vi "BioDaq_labview.vi"() -> ()   [LabVIEW 2013]
doc: "This example performs writes and reads on a serial port, as directed by the user. You can press the Write and Read buttons, and change the Read Count, while the example is running.\n\nThe parameters set for the serial port must match the parameters of the connected instrument or device. In this example, the Read Count parameter specifies the number of bytes that the serial port reads. If there were more bytes at the port than the specified number, those bytes would not be read. If there were less bytes at the port than the specified number, you would receive a timeout error.\n\nThis example expands upon the flow control options for XON and XOFF, allowing the user to choose those control characters. Also, the user can enable or disable a termination character. Some devices require a termination character in order to identify the end of command strings. Some devices send a termination character to signify the end of data to be read. This example shows how you can end the Read operation once a termination character is detected in the buffer and/or append a termination character at the end of the Write data."
uses:
  Program Files/National Instruments/LabVIEW 2013/examples/Instrument IO/Serial/support/Serial - Settings.ctl
  <vilib>/Instr/_visa.llb/VISA Configure Serial Port (Instr).vi
panel:
  in  "Write 8":bool
  in  "Write 7":bool
  in  "Write 6":bool
  in  "Write 5":bool
  out "device 4":bool
  out "device 3":bool
  out "Waveform Chart 9":T1(graph)
  out "Waveform Chart 8":T1(graph)
  out "Waveform Chart 7":T1(graph)
  out "unit type 3":dbl
  out "time3":dbl
  in  "Write 4":bool
  in  "Write 3":bool
  out "goniometer":u8(knob) scale=0.0..255.0
  out "unit type":dbl
  out "Waveform Chart 6":T1(graph)
  out "Waveform Chart 5":T1(graph)
  out "Waveform Chart 4":T1(graph)
  out "unit type 2":dbl
  out "time 2":dbl
  out "device 2":bool
  out "device 1":bool
  out "time":dbl
  in  "Write 2":bool
  out "Waveform Chart 3":T1(graph)
  out "Waveform Chart 2":T1(graph)
  out "Waveform Chart":T1(graph)
  in  "Stop":bool
  in  "Command":string="*IDN?"
  in  "Write":bool
  in  "Serial Settings":T2={"baud rate"=115200, "data bits"=8, "parity"=enum."None", "stop bits"=10, "flow control"=0} {"flow control" items=["None"=0, "XON/XOFF"=1, "RTS/CTS"=2, "DTR/DSR"=4]; "stop bits" items=["1.0"=10, "1.5"=15, "2.0"=20]; "data bits" min=5 max=8 step=1; "baud rate" items=["75"=75, "110"=110, "134"=134, "150"=150, "300"=300, "600"=600, "1200"=1200, "1800"=1800, "2400"=2400, "4800"=4800, "7200"=7200, "9600"=9600, "14400"=14400, "19200"=19200, "28800"=28800, "38400"=38400, "56000"=56000, "57600"=57600, "115200"=115200, "128000"=128000, "230400"=230400]}
  in  "VISA resource name":refnum<visa-resource-name>="COM4"
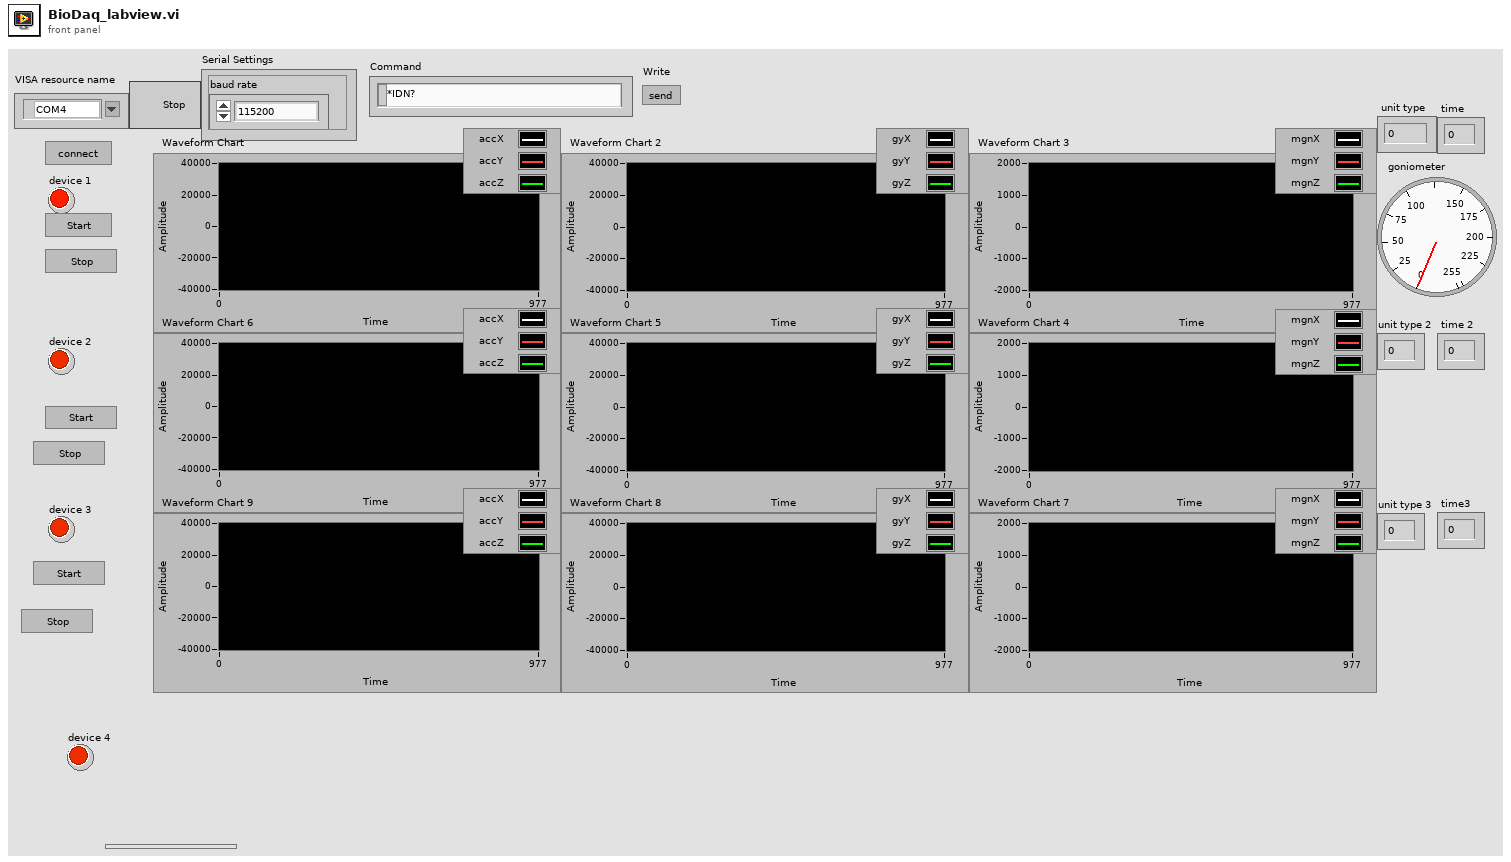
[diagram p1: front panel]
types:
  T1 = cluster{"Numeric Control":dbl, "Numeric Control":dbl, "Numeric Control":dbl}
  T2 = typedef "Serial - Settings.ctl" = cluster{"baud rate":u32, "data bits":u16, "parity":enum16{"None", "Odd", "Even", "Mark", "Space"}, "stop bits":u16, "flow control":u16}
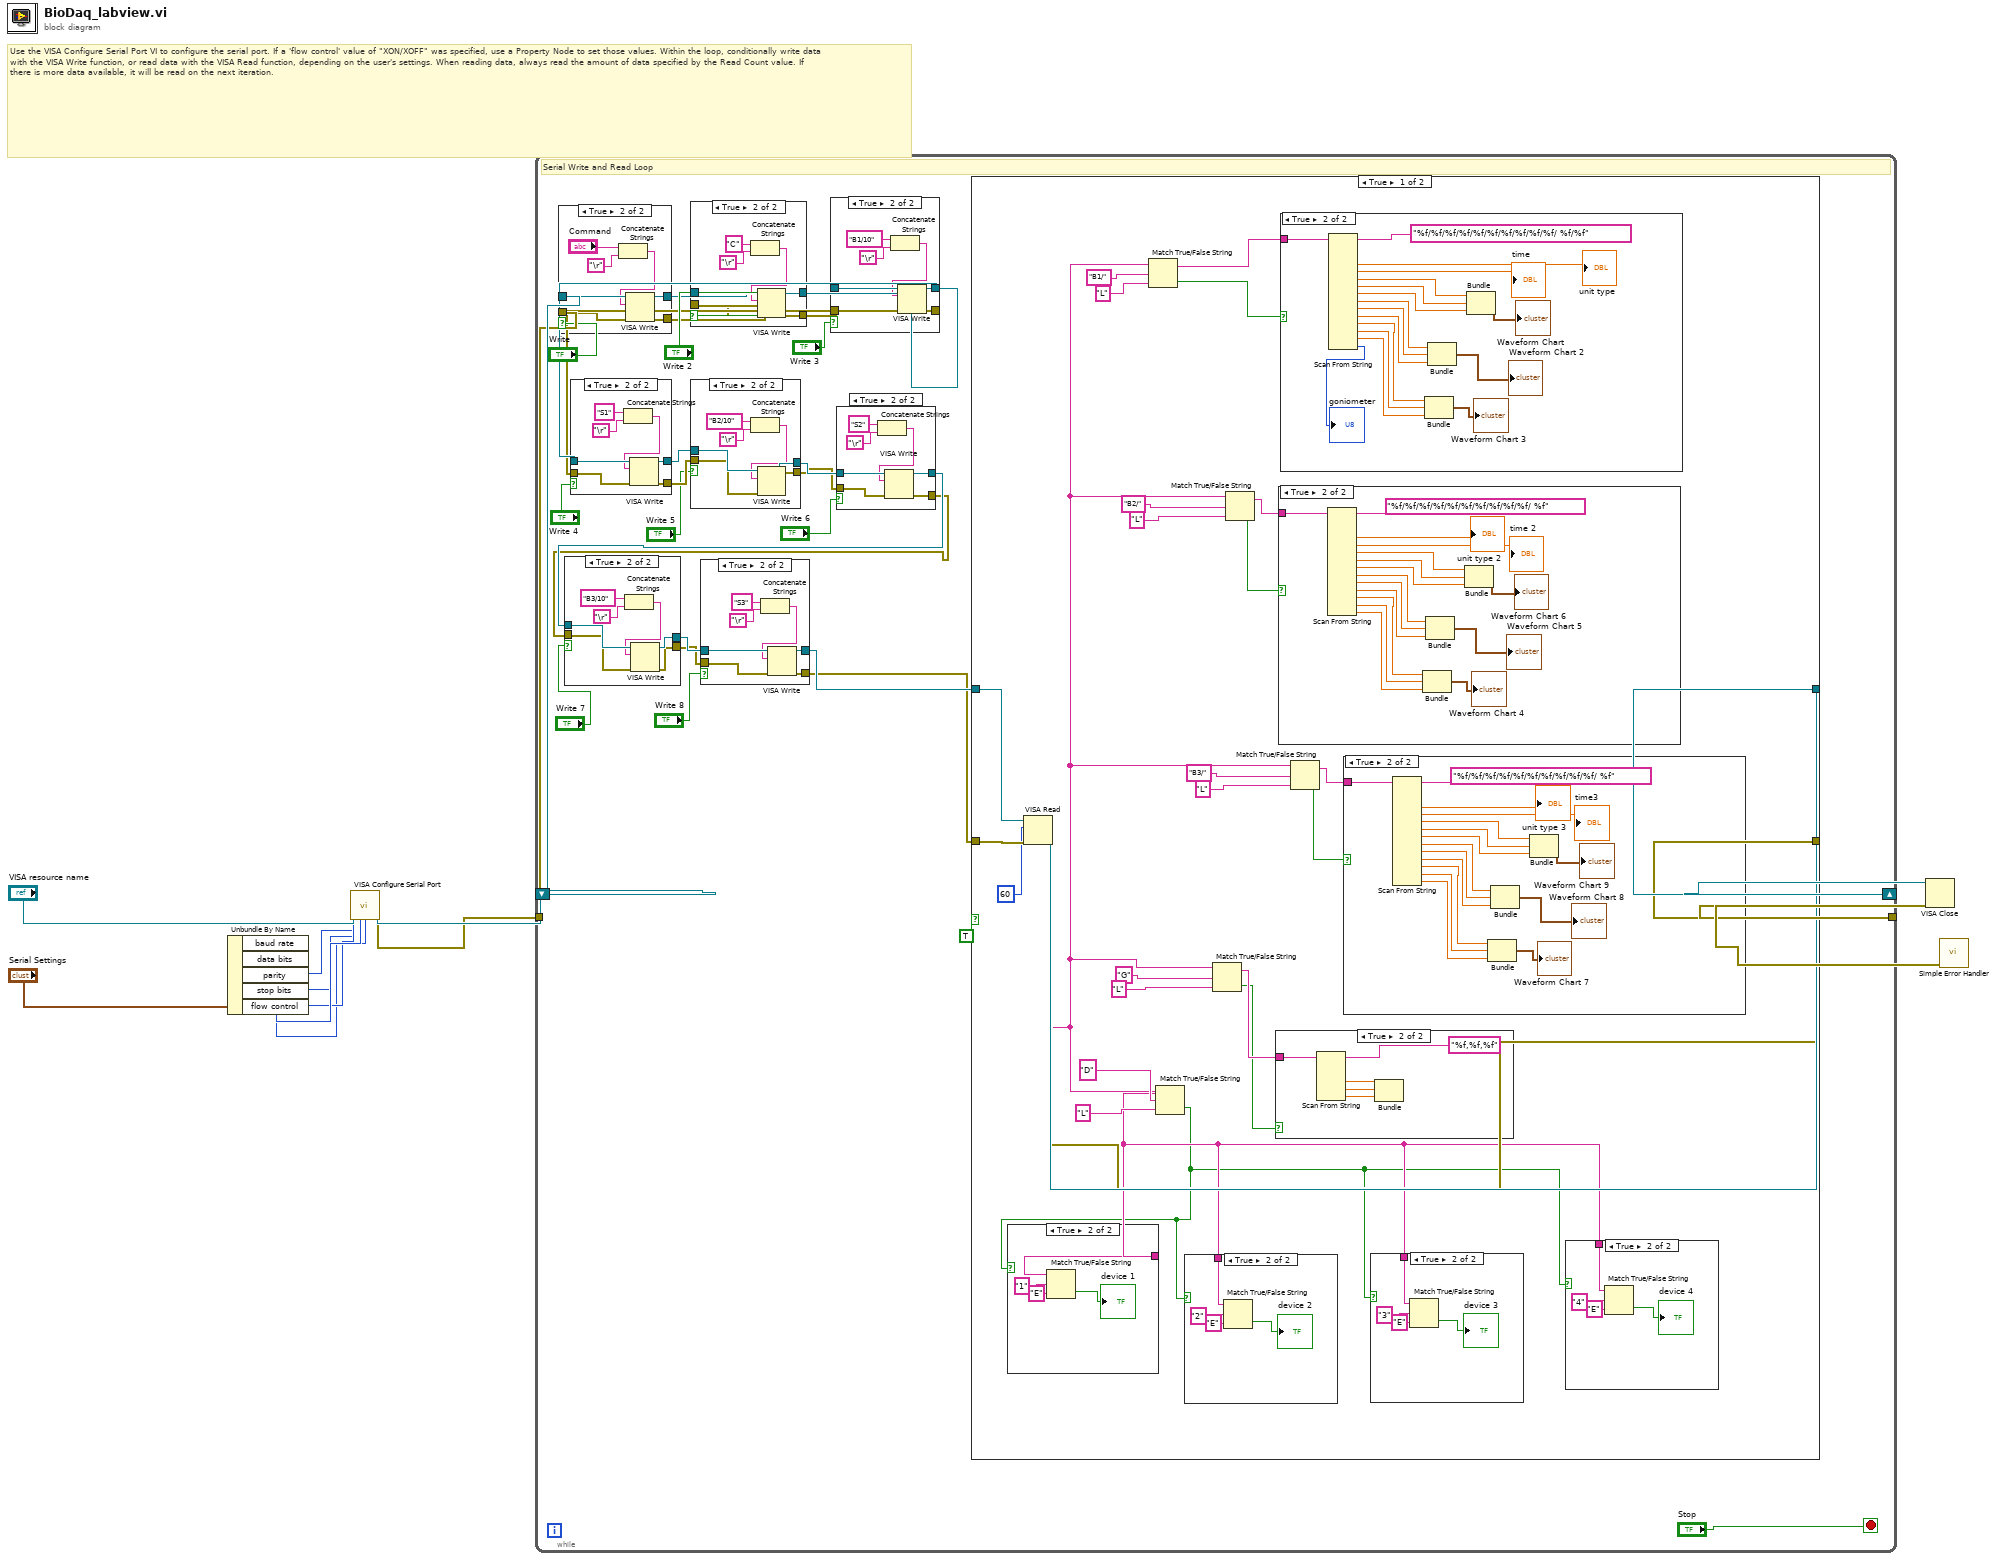
[diagram p0: block diagram]
diagram:
  # "Use the VISA Configure Serial Port VI to configure the serial port. If a 'flow control' value of \"XON/XOFF\" was specified, use a Property Node to set those values. Within the loop, conditionally write data with the VISA Write function, or read data with the VISA Read function, depending on the user's settings. When reading data, always read the amount of data specified by the Read Count value. If there is more data available, it will be read on the next iteration."
  n1 = Unbundle By Name("Serial Settings") -> ("baud rate"=w8:u32, "data bits"=w9:u16, "parity"=w10:enum16{"None", "Odd", "Even", "Mark", "Space"}, "stop bits"=w11:u16, "flow control"=w3:u16)
  n2 = call-poly "VISA Configure Serial Port"("VISA resource name"="VISA resource name", "baud rate (9600)"=w8, "data bits (8)"=w9, "parity (0:none)"=w10, "stop bits (10: 1 bit)"=w11, "flow control (0:none)"=w3) -> ("VISA resource name out"=w2:refnum<visa-resource-name>, "error out"=w1:errorcluster)  [unwired: 4 in, 4 out]
  n3 = while {
    shift-right: [w42] -> w4
    shift-left: w2 -> [w41]
    tunnel: w1 -> [w40]
    tunnel: [w39] -> w5
    stop <- "Stop" stop-if-true
    # "Serial Write and Read Loop"
    n4 = case shown="True" "Write" {
      tunnel: w41 -> [w107 w114]
      tunnel: w40 -> [w106 w113]
      tunnel: [w107 w112] -> w35
      tunnel: [w106 w111] -> w31
      frame False {
      }
      frame True {
        n5 = Concatenate Strings("Command", "\r") -> (w109:string)
        n6 = VISA Write(VISA resource name=w114, write buffer=w109, error in (no error)=w113) -> (VISA resource name out=w112:refnum<visa-resource-name>, error out=w111:errorcluster)  [unwired: 1 out]
      }
    }
    n7 = case shown="True" "Write 2" {
      tunnel: w35 -> [w98 w105]
      tunnel: w31 -> [w97 w100]
      tunnel: [w98 w104] -> w27
      tunnel: [w97 w103] -> w32
      frame False {
      }
      frame True {
        n8 = Concatenate Strings("C" ("string"), "\r") -> (w102:string)
        n9 = VISA Write(VISA resource name=w105, write buffer=w102, error in (no error)=w100) -> (VISA resource name out=w104:refnum<visa-resource-name>, error out=w103:errorcluster)  [unwired: 1 out]
      }
    }
    n10 = case shown="True" "Write 3" {
      tunnel: w27 -> [w89 w96]
      tunnel: w32 -> [w88 w91]
      tunnel: [w89 w95] -> w29
      tunnel: [w88 w94] -> w28
      frame False {
      }
      frame True {
        n11 = Concatenate Strings("B1/10" ("string"), "\r") -> (w93:string)
        n12 = VISA Write(VISA resource name=w96, write buffer=w93, error in (no error)=w91) -> (VISA resource name out=w95:refnum<visa-resource-name>, error out=w94:errorcluster)  [unwired: 1 out]
      }
    }
    n13 = case shown="True" "Write 4" {
      tunnel: w29 -> [w80 w87]
      tunnel: w28 -> [w79 w82]
      tunnel: [w80 w86] -> w26
      tunnel: [w79 w85] -> w25
      frame False {
      }
      frame True {
        n14 = Concatenate Strings("S1" ("string"), "\r") -> (w84:string)
        n15 = VISA Write(VISA resource name=w87, write buffer=w84, error in (no error)=w82) -> (VISA resource name out=w86:refnum<visa-resource-name>, error out=w85:errorcluster)  [unwired: 1 out]
      }
    }
    n16 = case shown="True" "Write 5" {
      tunnel: w26 -> [w71 w78]
      tunnel: w25 -> [w70 w73]
      tunnel: [w71 w77] -> w24
      tunnel: [w70 w76] -> w23
      frame False {
      }
      frame True {
        n17 = Concatenate Strings("B2/10" ("string"), "\r") -> (w75:string)
        n18 = VISA Write(VISA resource name=w78, write buffer=w75, error in (no error)=w73) -> (VISA resource name out=w77:refnum<visa-resource-name>, error out=w76:errorcluster)  [unwired: 1 out]
      }
    }
    n19 = case shown="True" "Write 6" {
      tunnel: w24 -> [w53 w60]
      tunnel: w23 -> [w52 w55]
      tunnel: [w53 w59] -> w18
      tunnel: [w52 w58] -> w17
      frame False {
      }
      frame True {
        n20 = Concatenate Strings("S2" ("string"), "\r") -> (w57:string)
        n21 = VISA Write(VISA resource name=w60, write buffer=w57, error in (no error)=w55) -> (VISA resource name out=w59:refnum<visa-resource-name>, error out=w58:errorcluster)  [unwired: 1 out]
      }
    }
    n22 = case shown="True" "Write 7" {
      tunnel: w18 -> [w62 w69]
      tunnel: w17 -> [w61 w64]
      tunnel: [w62 w68] -> w20
      tunnel: [w61 w67] -> w19
      frame False {
      }
      frame True {
        n23 = Concatenate Strings("B3/10" ("string"), "\r") -> (w66:string)
        n24 = VISA Write(VISA resource name=w69, write buffer=w66, error in (no error)=w64) -> (VISA resource name out=w68:refnum<visa-resource-name>, error out=w67:errorcluster)  [unwired: 1 out]
      }
    }
    n25 = case shown="True" "Write 8" {
      tunnel: w20 -> [w44 w51]
      tunnel: w19 -> [w43 w46]
      tunnel: [w44 w50] -> w16
      tunnel: [w43 w49] -> w15
      frame False {
      }
      frame True {
        n26 = Concatenate Strings("S3" ("string"), "\r") -> (w48:string)
        n27 = VISA Write(VISA resource name=w51, write buffer=w48, error in (no error)=w46) -> (VISA resource name out=w50:refnum<visa-resource-name>, error out=w49:errorcluster)  [unwired: 1 out]
      }
    }
    n28 = case shown="True" TRUE {
      tunnel: [w138 w212] -> w42
      tunnel: w16 -> [w140 w212]
      tunnel: [w135 w211] -> w39
      tunnel: w15 -> [w139 w211]
      frame True {
        n29 = VISA Read(VISA resource name=w140, byte count=u32 60, error in (no error)=w139) -> (VISA resource name out=w138:refnum<visa-resource-name>, read buffer=w117:string, error out=w135:errorcluster)  [unwired: 1 out]
        n30 = Match True/False String(2:"L" ("false string"), 3:"B1/" ("true string"), 4:w117) -> (0:w127:bool, 1:w128:string)
        n31 = Match True/False String(2:"L" ("false string"), 3:"D" ("true string"), 4:w117) -> (0:w115:bool, 1:w116:string)
        n32 = case shown="True" w115 {
          tunnel: w116 -> [_ w205]
          frame False {
          }
          frame True {
            n33 = Match True/False String(2:"E" ("false string"), 3:"1" ("true string"), 4:w205) -> (0:→"device 1":bool)  [unwired: 1 out]
          }
        }
        n34 = case shown="True" w115 {
          tunnel: w116 -> [_ w199]
          frame False {
          }
          frame True {
            n35 = Match True/False String(2:"E" ("false string"), 3:"2" ("true string"), 4:w199) -> (0:→"device 2":bool)  [unwired: 1 out]
          }
        }
        n36 = Match True/False String(2:"L" ("false string"), 3:"G" ("true string"), 4:w117) -> (0:w129:bool, 1:w130:string)
        n37 = Match True/False String(2:"L" ("false string"), 3:"B2/" ("true string"), 4:w117) -> (0:w123:bool, 1:w124:string)
        n38 = case shown="True" w129 {
          tunnel: w130 -> [_ w206]
          frame False {
          }
          frame True {
            n39 = Scan From String(format string="%f,%f,%f", input string=w206) -> (output 1=w209:dbl, output 2=w208:dbl, output 3=w207:dbl)  [unwired: 5 in, 3 out]
            n40 = Bundle(w209, w208, w207) -> ()  [unwired: 1 in, 1 out]
          }
        }
        n41 = case shown="True" w123 {
          tunnel: w124 -> [_ w194]
          frame False {
          }
          frame True {
            n42 = Scan From String(format string="%f/%f/%f/%f/%f/%f/%f/%f/%f/%f/ %f", input string=w194) -> (output 1=→"unit type 2":dbl, output 2=→"time 2":dbl, output 3=w193:dbl, output 4=w192:dbl, output 5=w191:dbl, output 6=w190:dbl, output 7=w189:dbl, output 8=w188:dbl, output 9=w186:dbl, output 10=w185:dbl, output 11=w184:dbl)  [unwired: 13 in, 3 out]
            n43 = Bundle(w186, w185, w184) -> (→"Waveform Chart 4":cluster{dbl, dbl, dbl})  [unwired: 1 in]
            n44 = Bundle(w190, w189, w188) -> (→"Waveform Chart 5":cluster{dbl, dbl, dbl})  [unwired: 1 in]
            n45 = Bundle(w193, w192, w191) -> (→"Waveform Chart 6":cluster{dbl, dbl, dbl})  [unwired: 1 in]
          }
        }
        n46 = case shown="True" w127 {
          tunnel: w128 -> [_ w167]
          frame False {
          }
          frame True {
            n47 = Scan From String(format string="%f/%f/%f/%f/%f/%f/%f/%f/%f/%f/ %f/%f", input string=w167) -> (output 1=→"unit type":dbl, output 2=→"time":dbl, output 3=w178:dbl, output 4=w177:dbl, output 5=w176:dbl, output 6=w175:dbl, output 7=w174:dbl, output 8=w173:dbl, output 9=w171:dbl, output 10=w170:dbl, output 11=w169:dbl, output 12=→"goniometer":u8)  [unwired: 14 in, 3 out]
            n48 = Bundle(w171, w170, w169) -> (→"Waveform Chart 3":cluster{dbl, dbl, dbl})  [unwired: 1 in]
            n49 = Bundle(w175, w174, w173) -> (→"Waveform Chart 2":cluster{dbl, dbl, dbl})  [unwired: 1 in]
            n50 = Bundle(w178, w177, w176) -> (→"Waveform Chart":cluster{dbl, dbl, dbl})  [unwired: 1 in]
          }
        }
        n51 = Match True/False String(2:"L" ("false string"), 3:"B3/" ("true string"), 4:w117) -> (0:w118:bool, 1:w119:string)
        n52 = case shown="True" w118 {
          tunnel: w119 -> [_ w161]
          frame False {
          }
          frame True {
            n53 = Scan From String(format string="%f/%f/%f/%f/%f/%f/%f/%f/%f/%f/ %f", input string=w161) -> (output 1=→"unit type 3":dbl, output 2=→"time3":dbl, output 3=w160:dbl, output 4=w159:dbl, output 5=w158:dbl, output 6=w157:dbl, output 7=w156:dbl, output 8=w155:dbl, output 9=w153:dbl, output 10=w152:dbl, output 11=w151:dbl)  [unwired: 13 in, 3 out]
            n54 = Bundle(w153, w152, w151) -> (→"Waveform Chart 7":cluster{dbl, dbl, dbl})  [unwired: 1 in]
            n55 = Bundle(w157, w156, w155) -> (→"Waveform Chart 8":cluster{dbl, dbl, dbl})  [unwired: 1 in]
            n56 = Bundle(w160, w159, w158) -> (→"Waveform Chart 9":cluster{dbl, dbl, dbl})  [unwired: 1 in]
          }
        }
        n57 = case shown="True" w115 {
          tunnel: w116 -> [_ w146]
          frame False {
          }
          frame True {
            n58 = Match True/False String(2:"E" ("false string"), 3:"3" ("true string"), 4:w146) -> (0:→"device 3":bool)  [unwired: 1 out]
          }
        }
        n59 = case shown="True" w115 {
          tunnel: w116 -> [_ w142]
          frame False {
          }
          frame True {
            n60 = Match True/False String(2:"E" ("false string"), 3:"4" ("true string"), 4:w142) -> (0:→"device 4":bool)  [unwired: 1 out]
          }
        }
      }
      frame False {
      }
    }
  }
  n61 = VISA Close(VISA resource name=w4, error in (no error)=w5) -> (error out=w6:errorcluster)
  n62 = call <vilib>:"Simple Error Handler.vi"("error in (no error)"=w6) -> ()  [unwired: 1 in, 8 out]
